vi "getWavelength_v80AM6.vi"() -> ()   [LabVIEW 2016]
uses:
  <vilib>/Analysis/baseanly.llb/Mean (DBL).vi
  x32/CLDevIFace.dll
  <vilib>/Analysis/NI_AALBase.lvlib
panel:
  out "Wavelength":dbl format="%0.5f"
  out "1ppmWave (nm)":dbl format="%#_3g"
  out "1ppmFreq (MHz)":dbl
  out "Freq (Hz)":dbl
  out "standard deviation":dbl format="%0.5f"
  in  "# for Stdev":i32=7
  in  "Avg":i32=1
  out "Delta MHz":dbl
  in  "Scale Factor":dbl=800.0
  out "Power (mW)":dbl format="%.9f"
  out "return type":i32
  in  "Clear Chart?":bool
  in  "Delay Time (s)":dbl=0.01
  out "XY Graph":cluster{i32[], dbl[]}(graph)
  out "error out":errorcluster
  out "output param":i32
  in  "stop":bool
  in  "OK Button":bool
  in  "CommPort":dbl=6.0 caption="Comm Port #"
  # "Super cavity FSR  6 GHz\nZerodure FSR  750 MHz"
  # "1 pm = 200 MHz @1212nm\n1 pm = 800 MHz @606 nm"
  # "Bristol 621B accuracy = 0.75 ppm\nuseful conversions:"
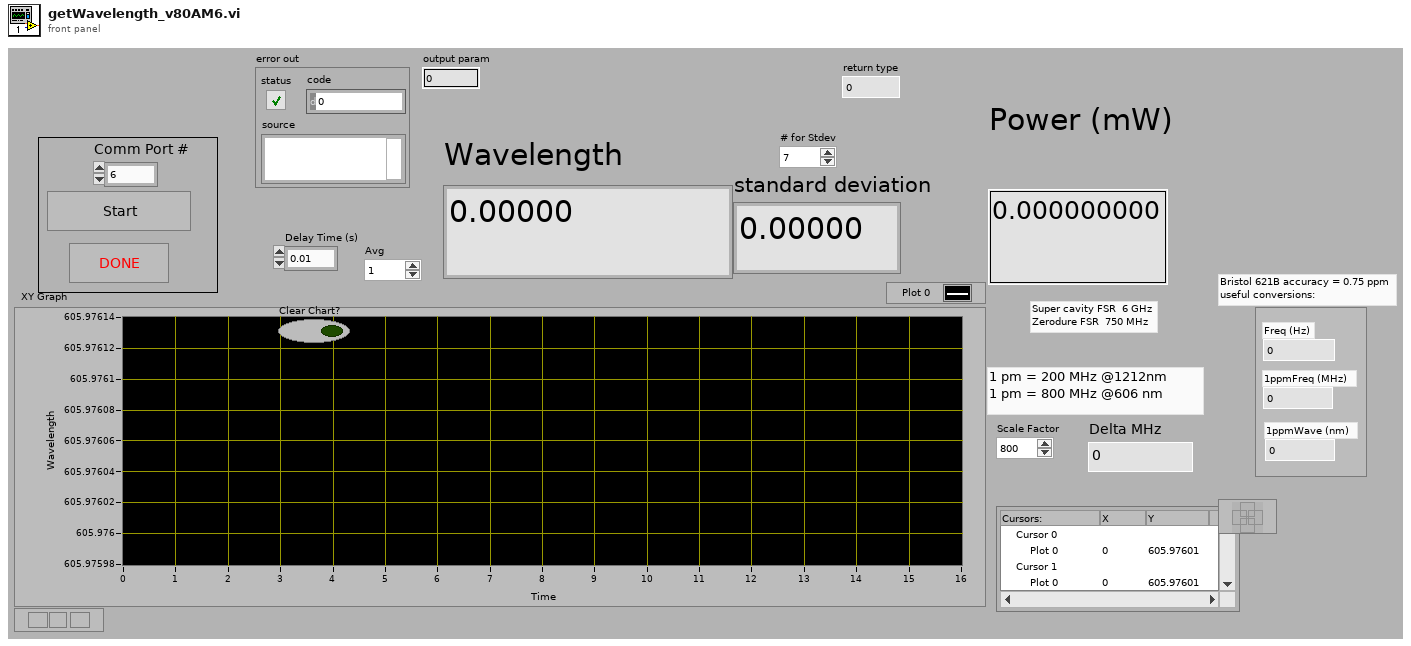
[diagram p1: front panel]
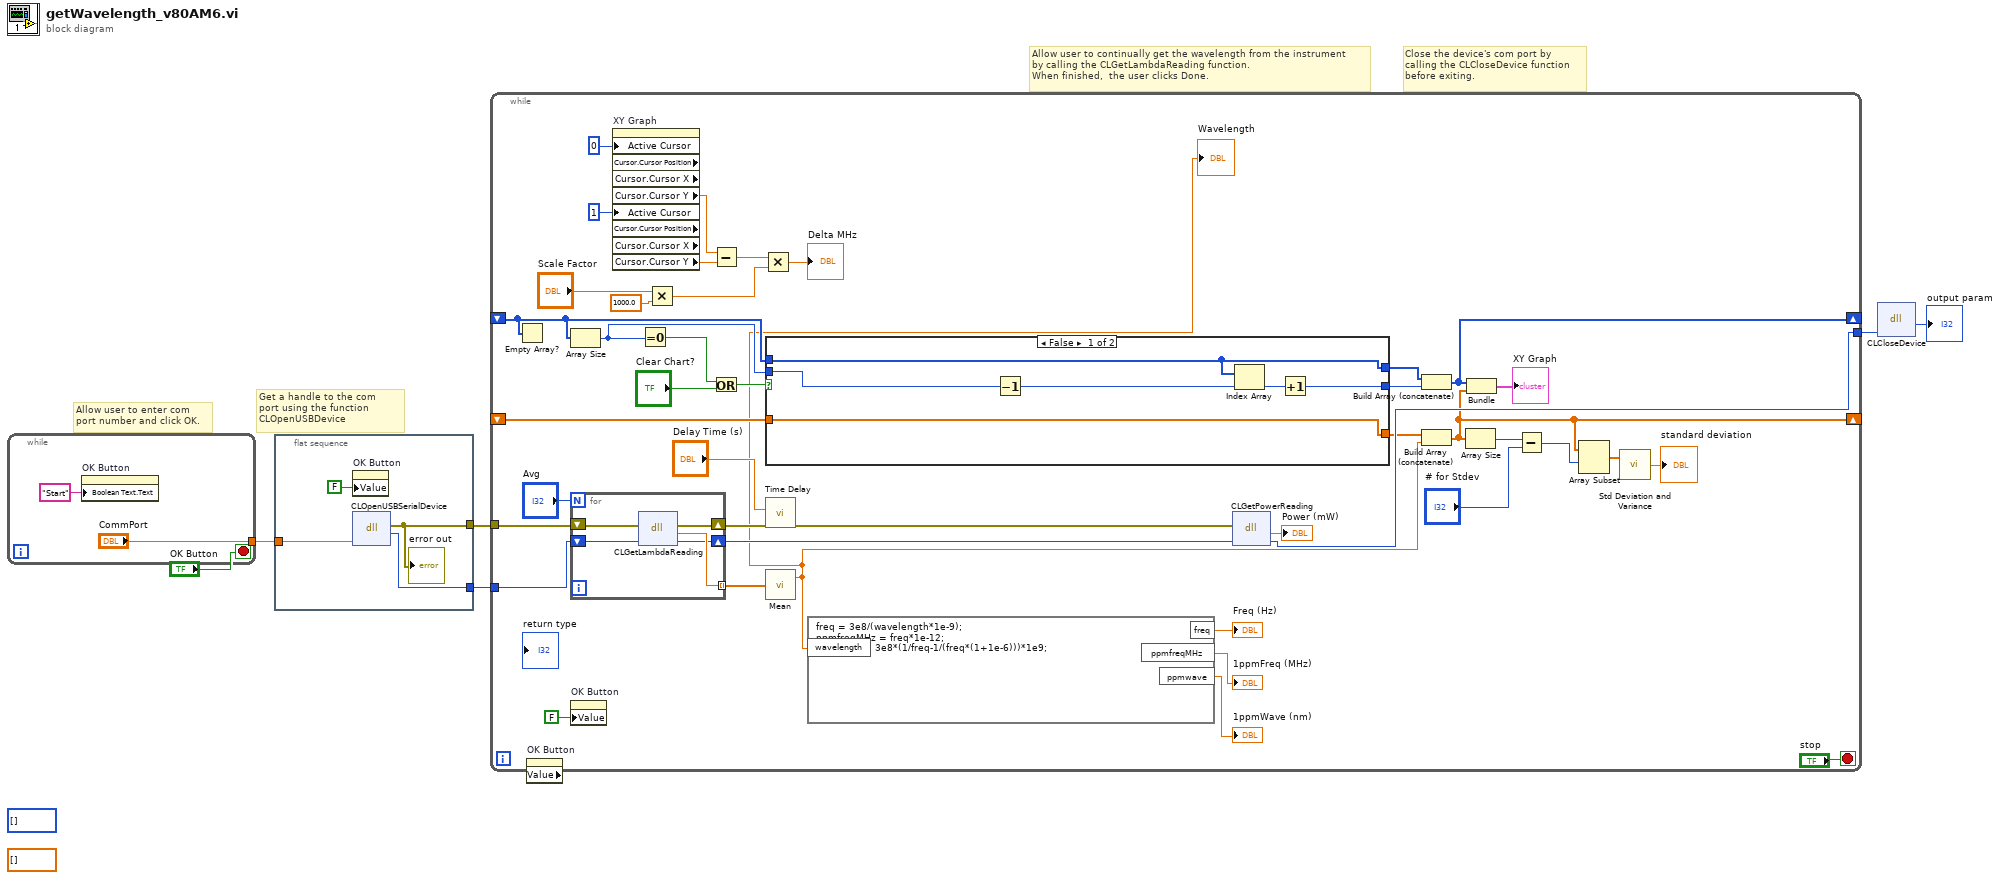
[diagram p0: block diagram]
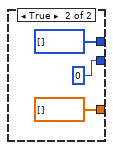
[diagram p2: hidden frame]
diagram:
  (unwired) i32[] []
  (unwired) dbl[] []
  # "Close the device's com port by\ncalling the CLCloseDevice function\nbefore exiting."
  # "Allow user to continually get the wavelength from the instrument\nby calling the CLGetLambdaReading function.  \nWhen finished,  the user clicks Done."
  # "Get a handle to the com\nport using the function CLOpenUSBDevice"
  # "Allow user to enter com \nport number and click OK."
  n1 = while {
    tunnel: ["CommPort"] -> w5
    stop <- "OK Button" stop-if-true
    n2 = property on="OK Button" class="Bool (strict)"("Boolean Text.Text"="Start") -> ()  [unwired: 2 in, 2 out]
  }
  n3 = flat-sequence {
    tunnel: w5 -> [w12]
    tunnel: [w11] -> w4
    tunnel: [w9] -> w1
    frame #0 {
      n4 = property on="OK Button" class="Bool (strict)"("Value"=FALSE) -> ()  [unwired: 2 in, 2 out]
      n5 = dll-call lib="C:/Users/Lab/Desktop/Bristol wavemeter 621/00424-2-00 621 customer CD/Programming Interface/x32/CLDevIface.dll" fn="CLOpenUSBSerialDevice"("commPort"=w12) -> (error out=w9:errorcluster, "return type"=w11:i32)  [unwired: 4 in, 1 out]
      "error out" <- w9
    }
  }
  n6 = while {
    tunnel: w4 -> [w54]
    tunnel: [w42] -> w3
    shift-right: [w22] -> _
    shift-left: _ -> [w46]
    shift-right: [w51] -> _
    shift-left: _ -> [w27]
    tunnel: w1 -> [w47]
    stop <- "stop" stop-if-true
    n7 = Empty Array?(array=w27) -> ()  [unwired: 1 out]
    n8 = property on="OK Button" class="Bool (strict)" props=["Value"]() -> ()  [unwired: 2 in, 3 out]
    n9 = Array Size(array=w27) -> (size(s)=w24:i32)
    n10 = for {
      N: "Avg" -> [_]
      tunnel: [w58] -> w25 mode=indexing
      shift-right: [w55] -> w43
      shift-left: w54 -> [w59]
      shift-right: [w57] -> w48
      shift-left: w47 -> [w56]
      n11 = dll-call lib="C:/Users/Lab/Desktop/Bristol wavemeter 621/00424-2-00 621 customer CD/Programming Interface/x32/CLDevIface.dll" fn="CLGetLambdaReading"(error in=w56, "devHandle"=w59) -> (error out=w57:errorcluster, "return type"=w58:dbl, "devHandle"=w55:i32)  [unwired: 2 in, 1 out]
    }
    n12 = property on="OK Button" class="Bool (strict)"("Value"=FALSE) -> ()  [unwired: 2 in, 2 out]
    n13 = property on="XY Graph" class="XYGraph (strict)" props=["Active Cursor", "Cursor", "Cursor Position", "Cursor", "Cursor X", "Cursor", "Cursor Y", "Active Cursor", "Cursor", "Cursor Position", "Cursor", "Cursor X", "Cursor", "Cursor Y"]("Active Cursor"=u32 0, "Active Cursor"=u32 1) -> ("Cursor.Cursor Y"=w38:dbl, "Cursor.Cursor Y"=w39:dbl)  [unwired: 2 in, 6 out]
    n14 = Equal To 0?(x=w24) -> (x = 0?=w32:bool)
    n15 = Multiply(x="Scale Factor", y=1000.0) -> (x*y=w33:dbl)
    n16 = Subtract(x=w38, y=w39) -> (x-y=w40:dbl)
    n17 = Or(x=w32, y="Clear Chart?") -> (x .or. y?=w30:bool)
    n18 = Multiply(x=w40, y=w33) -> (x*y=→"Delta MHz":dbl)
    n19 = case shown="False" w30 {
      tunnel: w46 -> [w65 _]
      tunnel: w27 -> [w64 _]
      tunnel: [w64 i32[] []] -> w28
      tunnel: [w65 dbl[] []] -> w29
      tunnel: w24 -> [w61 _]
      tunnel: [w62 0] -> w23
      frame False {
        n20 = Decrement(x=w61) -> (x-1=w60:i32)
        n21 = Index Array(array=w64, index=w60) -> (element=w63:i32)
        n22 = Increment(x=w63) -> (x+1=w62:i32)
      }
      frame True {
      }
    }
    n23 = call "Time Delay"("error in (no error)"=w48, "Delay Time (s)"="Delay Time (s)") -> ("error out"=w45:errorcluster)  [unwired: 9 in]
    n24 = call-poly <vilib>:"Mean.vi"("X"=w25) -> ("mean"=w13:dbl)  [unwired: 1 out]
    "Wavelength" <- w13
    n25 = formula code="freq = 3e8/(wavelength*1e-9);\nppmfreqMHz = freq*1e-12;\nppmwave = 3e8*(1/freq-1/(freq*(1+1e-6)))*1e9;"("wavelength"=w13) -> ("freq"=→"Freq (Hz)":dbl, "ppmfreqMHz"=→"1ppmFreq (MHz)":dbl, "ppmwave"=→"1ppmWave (nm)":dbl)
    n26 = dll-call lib="C:/Users/Lab/Desktop/Bristol wavemeter 621/00424-2-00 621 customer CD/Programming Interface/x32/CLDevIface.dll" fn="CLGetPowerReading"(error in=w45, "devHandle"=w43) -> ("return type"=→"Power (mW)":dbl, "devHandle"=w42:i32)  [unwired: 2 in, 2 out]
    n27 = Build Array (concatenate)(w28, w23) -> (w51:i32[])
    n28 = Build Array (concatenate)(w29, w13) -> (w22:dbl[])
    n29 = Array Size(array=w22) -> (size(s)=w21:i32)
    n30 = Bundle(w51, w22) -> (→"XY Graph":cluster{i32[], dbl[]})  [unwired: 1 in]
    n31 = Subtract(x=w21, y="# for Stdev") -> (x-y=w19:i32)
    n32 = Array Subset(array=w22, index=w19) -> (w18:dbl[])  [unwired: 1 in]
    n33 = call <vilib>:"Std Deviation and Variance.vi"("X"=w18) -> ("standard deviation"=→"standard deviation":dbl)  [unwired: 1 in, 2 out]
  }
  n34 = dll-call lib="C:/Users/Lab/Desktop/Bristol wavemeter 621/00424-2-00 621 customer CD/Programming Interface/x32/CLDevIface.dll" fn="CLCloseDevice"("commPort"=w3) -> ("return type"=→"output param":i32)  [unwired: 4 in, 2 out]
